vi "Build Custom Errors Section.vi"(8 "error in":errorcluster, 11 "Lv Proj Document Type:TAF Proj":refnum<class "Custom Errors.lvclass">) -> (0 "error out":errorcluster, 3 "Lv Proj Document Type:TAF Proj":refnum<class "Section.lvclass">)   [LabVIEW 2021, in "TAF Proj Document Type.lvlib" / "TAF Proj.lvclass"]
uses:
  <vilib>/Wovalab/AntiDoc/Document Type/Add-ons/LabVIEW TAF Project/TAF Proj/TAF Proj.lvclass
  <vilib>/Wovalab/AntiDoc/Section/Section.lvclass
  <vilib>/Wovalab/AntiDoc/Document Type/Add-ons/LabVIEW TAF Project/Custom Errors/Custom Errors.lvclass
  C:/Program Files (x86)/National Instruments/LabVIEW 2021/vi.lib/Wovalab/AntiDoc/Bloc/Bloc.lvclass
  <vilib>/Wovalab/AntiDoc/Document Type/Add-ons/LabVIEW TAF Project/Custom Errors/Custom Errors.lvclass/Custom Errors.ctl
  <vilib>/Wovalab/AntiDoc/Document Type/Add-ons/LabVIEW TAF Project/Custom Errors/Read Custom Errors.vi
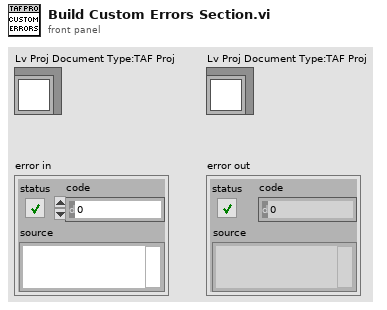
[diagram p1: front panel]
types:
  T1 = typedef "AntiDoc.lvlib/Bloc.lvclass/Custom Error Info--cluster.ctl" = cluster{"Code":i32, "Name":string, "Description":string, "Owned By":string[]}
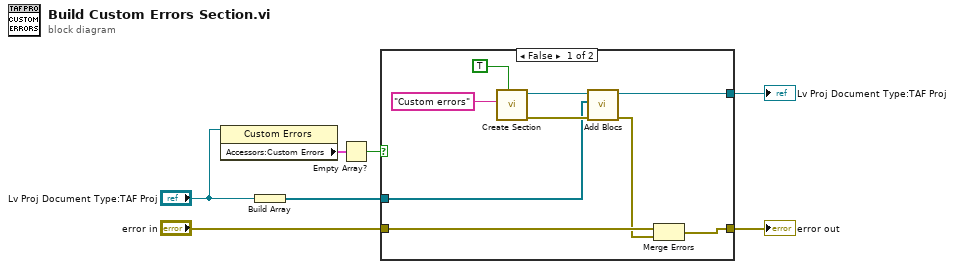
[diagram p0: block diagram]
diagram:
  n1 = property class="Custom Errors"(reference="Lv Proj Document Type:TAF Proj") -> ("Accessors:Custom Errors"=w2:T1[])  [unwired: 1 in, 2 out]
  n2 = Build Array("Lv Proj Document Type:TAF Proj") -> (w4:refnum<class "Custom Errors.lvclass">[])
  n3 = Empty Array?(array=w2) -> (empty?=w1:bool)
  n4 = case shown="False" w1 {
    tunnel: "error in" -> [w15 w17]
    tunnel: [w14 w17] -> w6
    tunnel: [w10 _] -> w5
    tunnel: w4 -> [w9 _]
    frame False {
      n5 = call <vilib>:"Create Section.vi"("No Title (F)"=TRUE, "Name"="Custom errors") -> ("error out"=w16:errorcluster, "Section out"=w12:refnum<class "Section.lvclass">)  [unwired: 8 in]
      n6 = call <vilib>:"Add Blocs.vi"("error in (no error)"=w16, "Blocs"=w9, "Section in"=w12) -> ("error out"=w13:errorcluster, "Section out"=w10:refnum<class "Section.lvclass">)  [unwired: 7 in]
      n7 = Merge Errors(w15, w13) -> (w14:errorcluster)
    }
    frame True {
    }
  }
  "Lv Proj Document Type:TAF Proj" <- w5
  "error out" <- w6
